vi "Graph - Silver FFT.vi"() -> ()   [LabVIEW 2011]
doc: "Sample numeric display item."
uses:
  <vilib>/NI Veristand/Display Template Support/Display Template Support.llb/cluster_Screen Item Settings.ctl
  <vilib>/NI Veristand/Display Template Support/Display Template Support.llb/cluster_Graph Scale Settings.ctl
  <vilib>/NI Veristand/Display Template Support/Display Template Support.llb/cluster_Graph Plot Settings.ctl
  <vilib>/NI Veristand/Display Template Support/Display Template Support.llb/cluster_Graph Handler Message.ctl
  <vilib>/NI Veristand/Display Template Support/Display Template Support.llb/enum_Graph Handler Message.ctl
  <vilib>/NI Veristand/Display Template Support/Display Template Support.llb/sub_Display Template Handler Graph.vi
  <vilib>/NI Veristand/Display Template Support/Display Template Support.llb/sub_Display Template Data Handler Graph.vi
  <vilib>/express/express analysis/Spectral/Block/exnSpectralBlock spectral measurements peak poly.vi
  <vilib>/express/express analysis/Spectral/Block/exnSpectralBlock spectral measurements peak array WFM.vi
  <vilib>/express/express analysis/Spectral/XNode/ExpressSpectralMeasurementsBlockNode.xnode
panel:
  in  "Local.Stop":bool
  out "Graph":cluster{"f0":dbl, "df":dbl, "magnitude":dbl[]}[](graph)
  out "Label":string="Numeric"
  in  "Save":bool
  out "Y.Autoscale":bool
  in  "Y.Scale.Once":bool
  in  "Y.Scale.Auto":bool
  out "X.Autoscale":bool
  in  "X.Scale.Once":bool
  in  "X.Scale.Auto":bool
  in  "Legend":bool
  in  "Setup":bool
  in  "Hold":bool
  in  "Item.Data":T1
  # "Autoscale X"
  # "Autoscale Y"
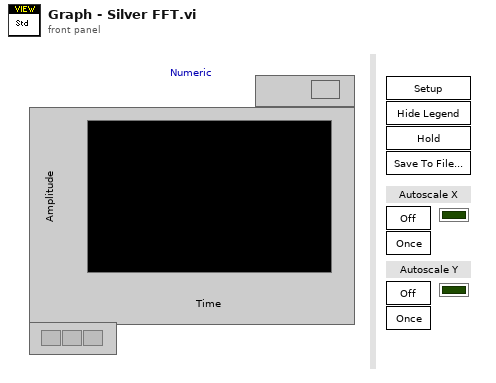
[diagram p1: front panel]
types:
  T1 = typedef "cluster_Screen Item Settings.ctl" = cluster{"Template VI":string, "Position X":i32, "Position Y":i32, "Custom":string, "Show Title Bar":bool, "ID":i32, "Always On Top":bool, "Allow Resize":bool, "Allow Minimize":bool, "Allow Close":bool, "Size to Screen":bool, "Screen.ID":i32, "State":enum16{"Normal", "New"}, "Title":string, "Window Bounds":cluster{"[0]":i16, "[1]":i16, "[2]":i16, "[3]":i16}, "Channel Ref":u64, "Unit":string, "Default Units?":bool, "Flash Limit?":bool, "Color 1":u32, "Color 2":u32, "Color 3":u32, "Color 4":u32, "Bck Color":u32, "Fore Color":u32, "Limit 1":dbl, "Limit 2":dbl, "Limit 3":dbl, "Limit 4":dbl, "Limit Mode 1":i32, "Limit Mode 2":i32, "Limit Mode 3":i32, "Limit Mode 4":i32, "Scale Precision":i32, "Scale Min":dbl, "Scale Max":dbl, "Format":i32, "Precision":i32, "Background Type":i32, "IDs":i32[], "Units":string[], "Labels":string[], "Scale Factor":dbl, "Scale Offset":dbl, "YScale Index":u32[], "XScale":T2, "YScales":T2[], "Plots":T3[], "Update Period":dbl, "History Length":dbl, "My.Ref":refnum<vi>, "Is Control?":bool, "Channel Paths":string[], "Custom Data":variant}
  T2 = typedef "cluster_Graph Scale Settings.ctl" = cluster{"Format":u8, "Precision":u8, "Fit":u8, "Label":string, "Use Default Label":bool, "Label Visible":bool, "Min":dbl, "Max":dbl}
  T3 = typedef "cluster_Graph Plot Settings.ctl" = cluster{"Bar Style":u8, "Fill To":i16, "Fill/PtColor":u32, "Line Style":u8, "Line Width":u8, "Color":u32, "Interp":u8, "Point Style":u8}
  T4 = cluster{"Command":enum16{"None", "Save"}, "Data":dbl[][]}
  T5 = typedef "cluster_Graph Handler Message.ctl" = cluster{"Message":T6, "Data":variant}
  T6 = typedef "enum_Graph Handler Message.ctl" = enum16{"None", "Stop", "Hold", "Update Channels", "New Settings", "Control Value", "Edit Value"}
  T7 = cluster{"averaging mode":u16, "weighting mode":u16, "number of averages":u32}
  T8 = cluster{"dB On (F)":bool, "unwrap phase (F)":bool, "convert to degree (F)":bool}
  T9 = enum16{"open", "replace", "create", "open or create", "replace or create", "replace or create with confirmation"}
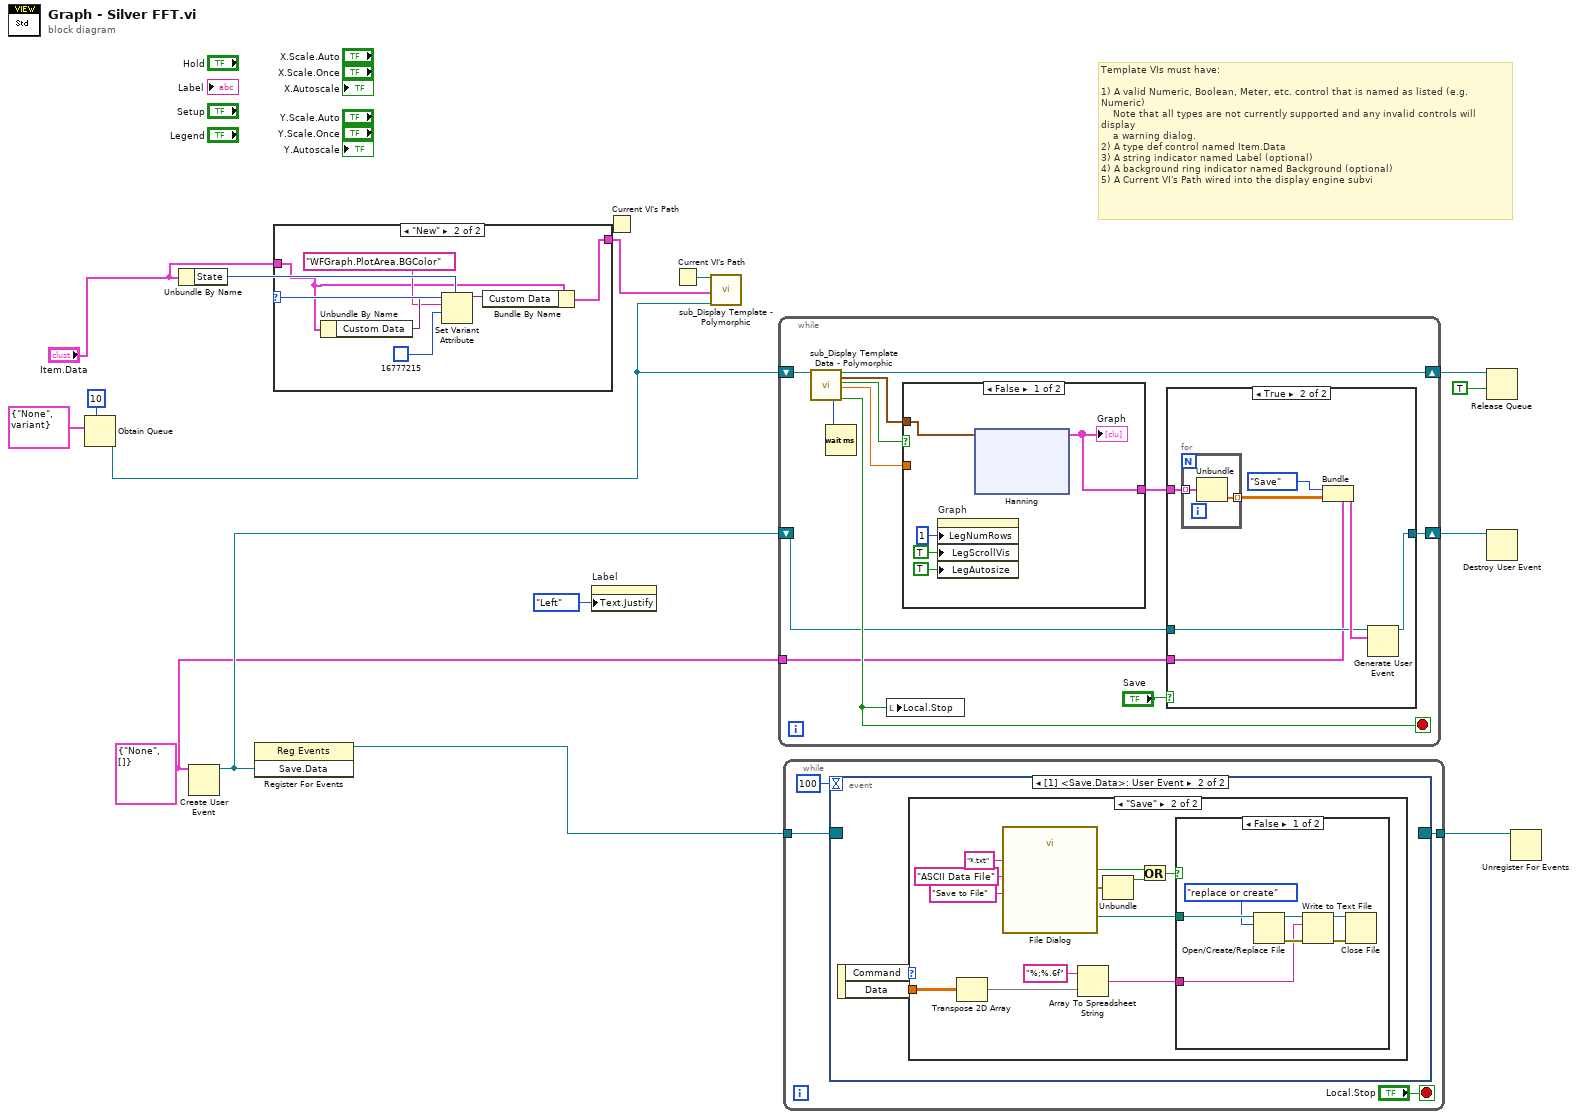
[diagram p0: block diagram]
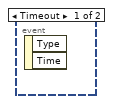
[diagram p3: hidden frame]
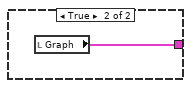
[diagram p7: hidden frame]
diagram:
  w5 = T4 {"Command"=enum."None", "Data"=[]} ("Save.Data")
  # "Template VIs must have:\n\n1) A valid Numeric, Boolean, Meter, etc. control that is named as listed (e.g. Numeric)\n    Note that all types are not currently supported and any invalid controls will display\n    a warning dialog.\n2) A type def control named Item.Data\n3) A string indicator named Label (optional)\n4) A background ring indicator named Background (optional)\n5) A Current VI's Path wired into the display engine subvi"
  n1 = Obtain Queue(max queue size (-1, unlimited)=10, element data type=T5 {"Message"=enum."None", "Data"=variant} ("Message")) -> (queue out=w10:refnum<queue>)  [unwired: 2 in, 3 out]
  n2 = Unbundle By Name("Item.Data") -> ("State"=w4:enum16{"Normal", "New"})
  n3 = Create User Event(user event datatype=w5) -> (user event=w9:refnum<user-event>)  [unwired: 1 in, 1 out]
  n4 = register-events(w9) -> (reference out=w8:refnum<event-registration>)  [unwired: 2 in, 1 out]
  n5 = case shown="\"New\"" w4 {
    tunnel: "Item.Data" -> [w16 w18]
    tunnel: [w16 w17] -> w2
    frame "Normal", Default {
    }
    frame "New" {
      n6 = Unbundle By Name(w18) -> ("Custom Data"=w22:variant)
      n7 = Set Variant Attribute(Variant=w22, name="WFGraph.PlotArea.BGColor", value=u32 16777215) -> (Variant out=w19:variant)  [unwired: 1 in, 2 out]
      n8 = Bundle By Name(cluster=w18, "Custom Data"=w19) -> (w17:T1)
    }
  }
  n9 = property on="Label" class="Str"("Text.Justify"=enum16{"Left", "Center", "Right"}."Left" ("Label.Justification")) -> ()  [unwired: 2 in, 2 out]
  n10 = Current VI's Path() -> ()  [unwired: 1 out]
  n11 = Current VI's Path() -> (path=w15:path)
  n12 = call-poly <vilib>:"sub_Display Template - Polymorphic.vi"("Parent.Path"=w15, "Item.Data"=w2, "queue"=w10) -> ()  [unwired: 17 out]
  n13 = while {
    shift-right: [w34] -> w14
    shift-left: w10 -> [w33]
    shift-right: [w29] -> w7
    shift-left: w9 -> [w26]
    tunnel: w5 -> [w23]
    stop <- w28 stop-if-true
    n14 = call-poly <vilib>:"sub_Display Template Data - Polymorphic.vi"("queue"=w33) -> ("Wait.Time"=w31:u32, "queue out"=w34:refnum<queue>, "Graph.Data"=w32:waveform(dbl)[], "Hold"=w24:bool, "XScale.Offset"=w25:dbl, "Stop"=w28:bool)  [unwired: 13 out]
    n15 = Wait (ms)(milliseconds to wait=w31) -> ()  [unwired: 1 out]
    n16 = local write "Local.Stop"(w28) -> ()
    n17 = case shown="False" w24 {
      tunnel: w25 -> [_ _]
      tunnel: w32 -> [w48 _]
      tunnel: [w49 w60] -> w27
      frame False {
        n18 = property on="Graph" class="WFGraph (strict)"("LegNumRows"=u32 1 ("Legend:Number of Rows"), "LegScrollVis"=TRUE ("Legend:Scrollbar Visible"), "LegAutosize"=TRUE ("Legend:Autosize")) -> ()  [unwired: 2 in, 2 out]
        n19 = xnode "Hanning"("Signals"=w48) -> ("FFT - (Peak)"=w49:cluster{"f0":dbl, "df":dbl, "magnitude":dbl[]}[])  [unwired: 1 in, 2 out]
        "Graph" <- w49
      }
      frame True {
        n20 = local read "Graph"() -> (w60:cluster{"f0":dbl, "df":dbl, "magnitude":dbl[]}[])
      }
    }
    n21 = case shown="True" "Save" {
      tunnel: [w35 w42] -> w29
      tunnel: w27 -> [_ w39]
      tunnel: w26 -> [w35 w37]
      tunnel: w23 -> [_ w36]
      frame False {
      }
      frame True {
        n22 = for {
          tunnel: w39 -> [w44] mode=indexing
          tunnel: [w43] -> w38 mode=indexing
          n23 = Unbundle(w44) -> ("magnitude"=w43:dbl[])  [unwired: 2 out]
        }
        n24 = Bundle(cluster=w36, "Command"=enum16{"None", "Save"}."Save", "Data"=w38) -> (w40:T4)
        n25 = Generate User Event(user event=w37, event data cluster=w40) -> (user event out=w42:refnum<user-event>)  [unwired: 1 in, 1 out]
      }
    }
  }
  n26 = while {
    tunnel: w8 -> [w64]
    tunnel: [w61] -> w6
    stop <- "Local.Stop" stop-if-true
    n27 = event shown="[1] <Save.Data>: User Event" {
      selector: w64 -> [_ _]
      dyn-events: [_ _] -> w61
      timeout: 100 -> [_ _]
      event Timeout {
        n28 = event-data() -> ()  [unwired: 3 out]
      }
      event User Event {
        n29 = event-data() -> ("Command"=w66:enum16{"None", "Save"}, "Data"=w65:dbl[][])  [unwired: 1 out]
        n30 = case shown="\"Save\"" w66 {
          tunnel: w65 -> [_ w68]
          frame "None", Default {
          }
          frame "Save" {
            n31 = Transpose 2D Array(2D array=w68) -> (transposed array=w67:dbl[][])
            n32 = call "File Dialog"("prompt"="Save to File", "pattern (all files)"="*.txt", "pattern label"="ASCII Data File") -> ("selected path"=w71:path, "cancelled"=w74:bool, "error out"=w75:errorcluster)  [unwired: 4 in, 6 out]
            n33 = Array To Spreadsheet String(array=w67, 3:"%;%.6f" ("format string")) -> (spreadsheet string=w69:string)  [unwired: 1 out]
            n34 = Unbundle(w75) -> ("status"=w73:bool)  [unwired: 2 out]
            n35 = Or(x=w74, y=w73) -> (x .or. y?=w72:bool)
            n36 = case shown="False" w72 {
              tunnel: w71 -> [w85 _]
              tunnel: w69 -> [w81 _]
              frame False {
                n37 = Open/Create/Replace File(file path (use dialog)=w85, operation (0:open)=T9."replace or create") -> (refnum out=w83:refnum<file>, error out=w82:errorcluster)  [unwired: 1 in, 4 out]
                n38 = Write to Text File(file (use dialog)=w83, text=w81, error in=w82) -> (refnum out=w80:refnum<file>, error out=w79:errorcluster)  [unwired: 2 out]
                n39 = Close File(refnum=w80, error in=w79) -> ()  [unwired: 2 out]
              }
              frame True {
              }
            }
          }
        }
      }
    }
  }
  n40 = Release Queue(queue=w14, force destroy? (F)=TRUE) -> ()  [unwired: 1 in, 3 out]
  n41 = Destroy User Event(user event=w7) -> ()  [unwired: 1 in, 1 out]
  n42 = Unregister For Events(event registration refnum=w6) -> ()  [unwired: 1 in, 1 out]
